vi "initilizeStates.vi"(8 "error in (no error)":errorcluster, 11 "guiTemplates in":refnum<class "stillnessHelper.lvclass">) -> (0 "error out":errorcluster, 3 "guiTemplates out":refnum<class "stillnessHelper.lvclass">)   [LabVIEW 2022 SP3, in "stillnessHelper.lvclass"]
uses:
  stillnessHelper.lvclass
  statesWithOptions.ctl
  stillnessHelper.lvclass/stillnessHelper.ctl
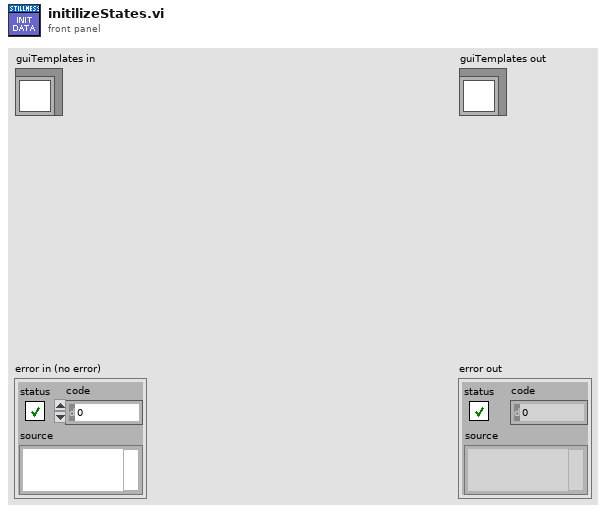
[diagram p1: front panel]
types:
  T1 = typedef "stillnessHelper.lvclass/statesWithOptions.ctl" = cluster{"States":string, "Options":string[]}
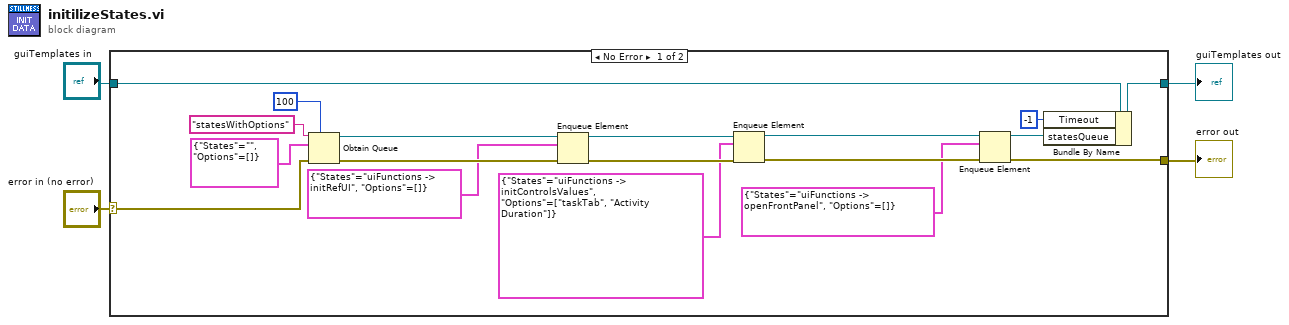
[diagram p0: block diagram]
diagram:
  n1 = case shown="No Error" "error in (no error)" {
    selector: "error in (no error)" -> [w17 w24]
    tunnel: [w6 w24] -> w3
    tunnel: [w15 w23] -> w1
    tunnel: "guiTemplates in" -> [w16 w23]
    frame No Error {
      n2 = Obtain Queue(max queue size (-1, unlimited)=100, name (unnamed)="statesWithOptions", element data type=T1 {"States"="", "Options"=[]} ("States WITH Options"), error in (no error)=w17) -> (queue out=w21:refnum<queue>, error out=w22:errorcluster)  [unwired: 1 in, 1 out]
      n3 = Enqueue Element(queue=w21, element=T1 {"States"="uiFunctions -> initRefUI", "Options"=[]} ("States WITH Options"), error in (no error)=w22) -> (queue out=w13:refnum<queue>, error out=w12:errorcluster)  [unwired: 1 in, 1 out]
      n4 = Enqueue Element(queue=w13, element=T1 {"States"="uiFunctions -> initControlsValues", "Options"=["taskTab", "Activity Duration"]} ("States WITH Options"), error in (no error)=w12) -> (queue out=w9:refnum<queue>, error out=w7:errorcluster)  [unwired: 1 in, 1 out]
      n5 = Enqueue Element(queue=w9, element=T1 {"States"="uiFunctions -> openFrontPanel", "Options"=[]} ("States WITH Options"), error in (no error)=w7) -> (queue out=w8:refnum<queue>, error out=w6:errorcluster)  [unwired: 1 in, 1 out]
      n6 = Bundle By Name(cluster=w16, "Timeout"=-1 ("State Machine Control.Timeout"), "statesQueue"=w8) -> (w15:refnum<class "stillnessHelper.lvclass">)
    }
    frame Error {
    }
  }
  "error out" <- w3
  "guiTemplates out" <- w1
